vi "Client Oven ON OFF.vi"() -> ()   [LabVIEW 2015]
uses:
  <vilib>/MakerHub/LINX/Public/Peripherals/Analog/Analog Read 1 Chan.vi
  <vilib>/MakerHub/LINX/Public/Peripherals/Digital/Digital Write 1 Chan.vi
  <vilib>/MakerHub/LINX/LMH-LINX.lvlib
panel:
  out "Error":dbl=1.0
  in  "dt":dbl=1.0
  in  "Setpoint":dbl=70.0
  out "Waveform Chart":cluster{"Setpoint":dbl, "Setpoint":dbl}(graph)
  in  "Connect":bool
  in  "About":bool
  in  "Stop":bool
  in  "VISA resource name":refnum<visa-resource-name>
  # "LabVIEW MakerHub"
  # "Proteus Test - Oven ON OFF"
  # "COM Port"
  # "Tmperature Plot"
  # "Quit"
  # "Error"
  # "Setpoint"
  # "dt"
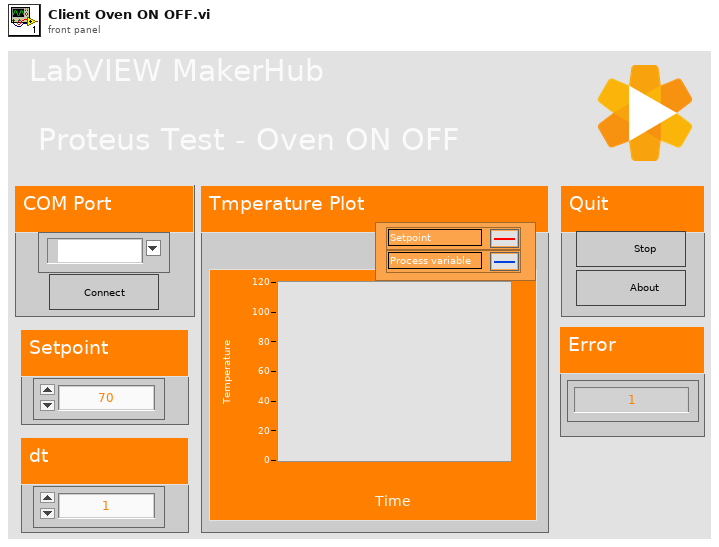
[diagram p1: front panel]
types:
  T1 = typedef "LMH-LINX.lvlib/LINX Ref.ctl" = cluster{"Platform":T2, "Interface":T3, "LINX Device Config":T4}
  T2 = typedef "LMH-LINX.lvlib/Platform.ctl" = enum16{"LINX", "myRIO"}
  T3 = typedef "LMH-LINX.lvlib/Interface.ctl" = enum16{"Serial", "TCP"}
  T4 = typedef "LMH-LINX.lvlib/Device.lvlib/LINX Device Config.ctl" = cluster{"Interface":T3, "COM Port":refnum<visa-resource-name>, "TCP Configuration":T5, "Device Family":u8, "Device ID":u8, "Device Name":string, "TCP Ref":refnum<k5>, "Channels":T6}
  T5 = typedef "LMH-LINX.lvlib/Device.lvlib/TCP Config.ctl" = cluster{"IP Address":string, "Port":u16}
  T6 = typedef "LMH-LINX.lvlib/Channels.ctl" = cluster{"DI":u8[], "DO":u8[], "AI":u8[], "AO":u8[], "PWM":u8[], "QE":u8[], "UART":u8[], "I2C 2":u8[], "SPI":u8[], "CAN":u8[], "Servo":u8[], "AI Ref (V)":dbl, "AO Ref (V)":dbl, "AO Resolution (Bits)":u8}
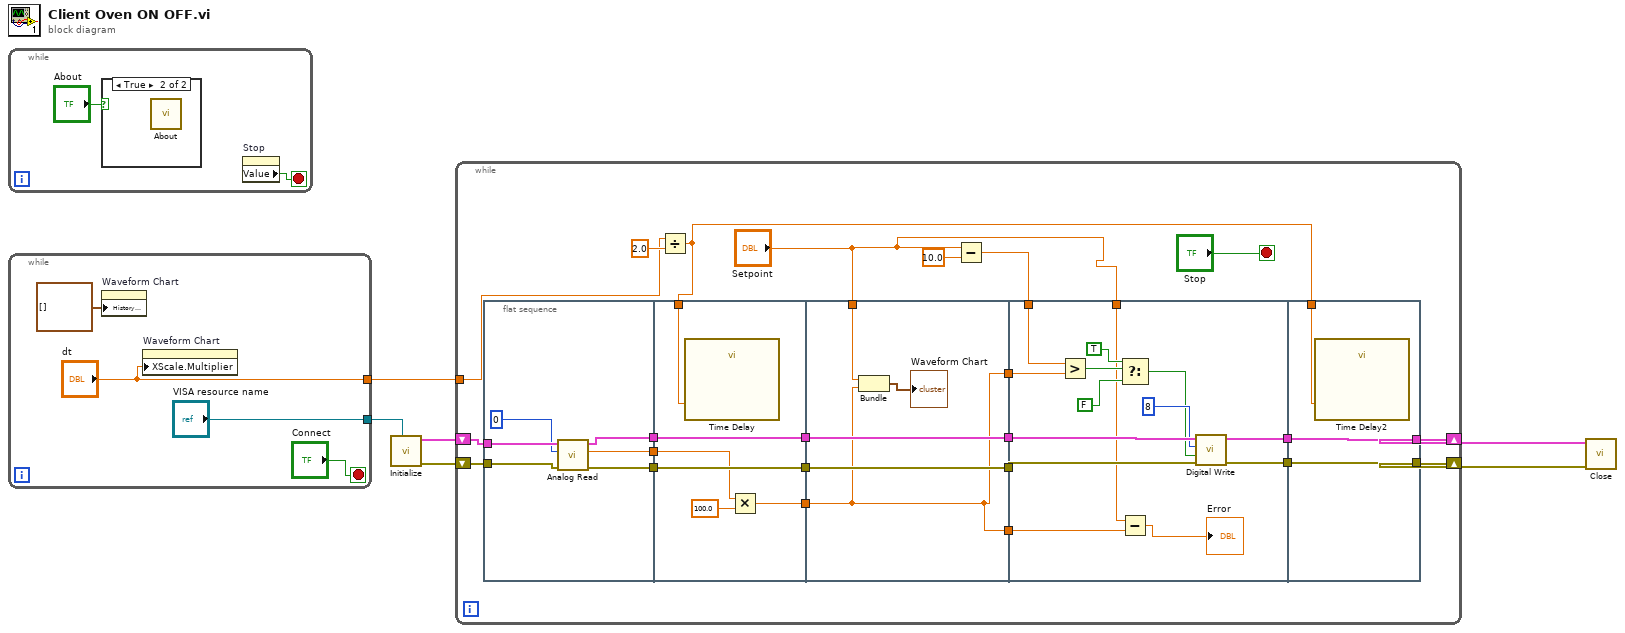
[diagram p0: block diagram]
diagram:
  n1 = while {
    stop <- w7 stop-if-true
    n2 = case shown="True" "About" {
      frame False {
      }
      frame True {
        n3 = call "About.vi"() -> ()  [unwired: 1 in]
      }
    }
    n4 = property on="Stop" class="Bool (strict)"() -> ("Value"=w7:bool)  [unwired: 2 in, 2 out]
  }
  n5 = while {
    tunnel: ["VISA resource name"] -> w6
    tunnel: ["dt"] -> w3
    stop <- "Connect" stop-if-true
    n6 = property on="Waveform Chart" class="WFChart (strict)"("History Data"=cluster{"Setpoint":dbl, "Setpoint":dbl}[] []) -> ()  [unwired: 2 in, 2 out]
    n7 = property on="Waveform Chart" class="WFChart (strict)"("XScale.Multiplier"="dt") -> ()  [unwired: 2 in, 2 out]
  }
  n8 = call <vilib>:"Initialize.vi"("Serial Port"=w6) -> ("Error Out"=w4:errorcluster, "LINX Ref"=w5:T1)  [unwired: 8 in, 1 out]
  n9 = while {
    shift-right: [w20] -> w2
    shift-left: w5 -> [w35]
    shift-right: [w18] -> w1
    shift-left: w4 -> [w34]
    tunnel: w3 -> [w28]
    stop <- "Stop" stop-if-true
    n10 = flat-sequence {
      tunnel: w35 -> [w41]
      tunnel: w34 -> [w40]
      tunnel: [w38] -> w32
      tunnel: [w37] -> w31
      tunnel: [w36] -> w30
      tunnel: w32 -> [w43]
      tunnel: w31 -> [w47]
      tunnel: w30 -> [w46]
      tunnel: w21 -> [w45]
      tunnel: [w47] -> w27
      tunnel: [w46] -> w26
      tunnel: [w42] -> w25
      tunnel: w27 -> [w52]
      tunnel: w26 -> [w51]
      tunnel: "Setpoint" -> [w49]
      tunnel: w25 -> [w48]
      tunnel: [w52] -> w24
      tunnel: [w51] -> w23
      tunnel: [w48] -> w22
      tunnel: [w48] -> w13
      tunnel: w24 -> [w65]
      tunnel: w23 -> [w66]
      tunnel: w15 -> [w59]
      tunnel: w22 -> [w58]
      tunnel: [w57] -> w19
      tunnel: [w56] -> w17
      tunnel: "Setpoint" -> [w54]
      tunnel: w13 -> [w53]
      tunnel: w21 -> [w69]
      tunnel: [w68] -> w20
      tunnel: w19 -> [w68]
      tunnel: [w67] -> w18
      tunnel: w17 -> [w67]
      frame #0 {
        n11 = call-poly <vilib>:"Analog Read.vi"("Error In"=w40, "Analog Channel"=u8 0, "LINX Resource"=w41) -> ("Error Out"=w37:errorcluster, "AI Value"=w38:dbl, "LINX Resource"=w36:T1)  [unwired: 5 in, 1 out]
      }
      frame #1 {
        n12 = call "Time Delay"("Delay Time (s)"=w45) -> ()  [unwired: 10 in, 1 out]
        n13 = Multiply(x=w43, y=100.0) -> (x*y=w42:dbl)
      }
      frame #2 {
        n14 = Bundle("Setpoint"=w49, w48) -> (→"Waveform Chart":cluster{"Setpoint":dbl, dbl})  [unwired: 1 in]
      }
      frame #3 {
        n15 = Greater?(x=w59, y=w58) -> (0:w61:bool)
        n16 = Select(t=TRUE, s=w61, f=FALSE) -> (s? t:f=w60:bool)
        n17 = Subtract(x=w54, y=w53) -> (x-y=→"Error":dbl)
        n18 = call-poly <vilib>:"Digital Write.vi"("Error In"=w65, "Output Value"=w60, "DO Channel"=8, "LINX Resource"=w66) -> ("Error Out"=w56:errorcluster, "LINX Resource"=w57:T1)  [unwired: 6 in]
      }
      frame #4 {
        n19 = call "Time Delay2"("Delay Time (s)"=w69) -> ()  [unwired: 10 in, 1 out]
      }
    }
    n20 = Divide(x=w28, y=2.0) -> (x/y=w21:dbl)
    n21 = Subtract(x="Setpoint", y=10.0) -> (x-y=w15:dbl)
  }
  n22 = call <vilib>:"Close.vi"("Error In"=w1, "LINX Resource"=w2) -> ()  [unwired: 8 in, 2 out]
